vi "data processor main.vi"(11 "dataProcessor":T1) -> ()   [LabVIEW 2018]
uses:
  type defs/data processor data.ctl
  type defs/channelLimitControl.ctl
  type defs/limitActions.ctl
  supporting VIs/polymorphic VIs/de-queue for data processor.vi
  supporting VIs/polymorphic VIs/enqueue for file IO.vi
  supporting VIs/polymorphic VIs/release data processor queue.vi
types:
  T1 = typedef "data processor data.ctl" = cluster{"params":cluster{"controlFeedback":cluster{"butterflyValue":u16, "ballValue":u16, "massflow":u16, "pressureRatio":u16, "compSpeed":u16}, "DAQrate":enum16{"50 kHz", "25 kHz", "16.6 kHz", "12.5 kHz", "10 kHz", "8.33 kHz", "7.14 kHz", "6.25 kHz", "5.55 kHz", "5 kHz"}, "safetyChannels":cluster{"oilP":u16, "airP":u16, "water":u16, "channelLimit":T2[]}, "channelConfigPath":path}, "vars":cluster{"controlFeedback":cluster{"butterflyValue":u16, "ballValue":u16, "massflow":u16, "pressureRatio":u16, "compSpeed":u16}, "activeChannelNames":string[], "activeChannelUnits":string[], "offset trigger":bool, "offsets":dbl[], "activeChannelLimitIndex":u16[], "liveData":bool}}
  T2 = typedef "channelLimitControl.ctl" = cluster{"channelID":u16, "Enabled":bool, "warnValue":dbl, "limitValue":dbl, "Invert":bool, "limitAction":T3}
  T3 = typedef "limitActions.ctl" = enum16{"stop", "shutdown", "ignore"}
  T4 = typedef "Queues.ctl" = cluster{"messageHandler":refnum<queue>, "comms":refnum<queue>, "dataStream":refnum<queue>, "dataProcessor":refnum<queue>, "fileIO":refnum<queue>, "userInterface":refnum<queue>, "errors":refnum<queue>, "customCompressor":refnum<queue>}
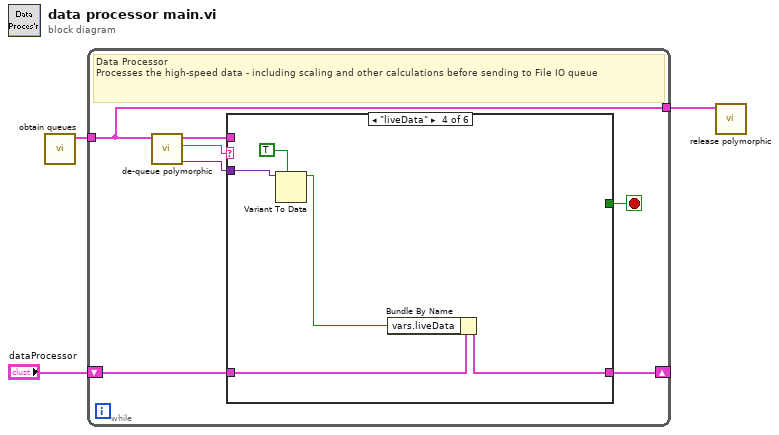
[diagram p0: block diagram]
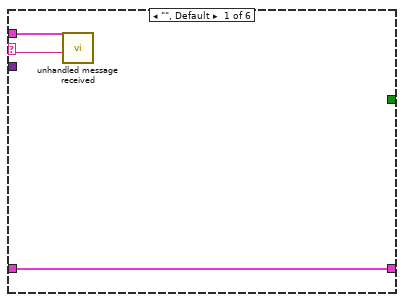
[diagram p2: hidden frame]
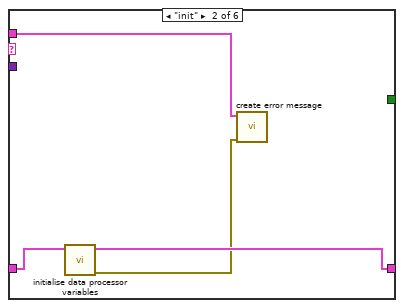
[diagram p3: hidden frame]
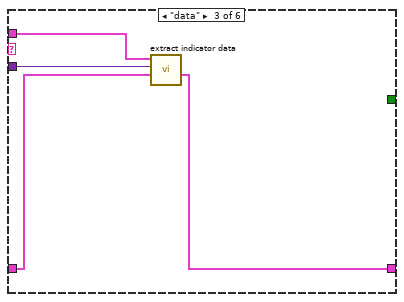
[diagram p4: hidden frame]
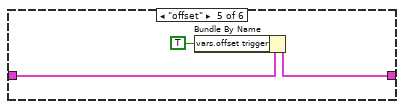
[diagram p5: hidden frame]
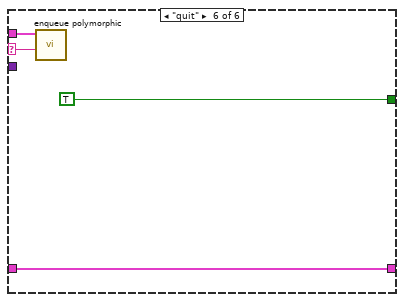
[diagram p6: hidden frame]
diagram:
  n1 = call "obtain queues.vi"() -> ("queues"=w2:T4)  [unwired: 11 in]
  n2 = while {
    tunnel: w2 -> [w6]
    tunnel: [w6] -> w1
    shift-right: [w5] -> _
    shift-left: "dataProcessor" -> [w4]
    stop <- w7 stop-if-true
    # "Data Processor\nProcesses the high-speed data - including scaling and other calculations before sending to File IO queue"
    n3 = call-poly "de-queue polymorphic.vi"("Queues"=w6) -> ("data"=w8:variant, "message"=w10:string, "Queues out"=w9:T4)  [unwired: 8 in]
    n4 = case shown="\"liveData\"" w10 {
      selector: w10 -> [w11 _ _ _ _ w32]
      tunnel: w9 -> [w12 w15 w19 _ _ w33]
      tunnel: w8 -> [_ _ w21 w25 _ _]
      tunnel: [_ _ _ _ _ TRUE] -> w7
      tunnel: [w13 w16 w18 w23 w28 w30] -> w5
      tunnel: w4 -> [w13 w17 w20 w26 w29 w30]
      frame "", Default {
        n5 = call "unhandled message received.vi"("unhandledMessage"=w11, "queues"=w12) -> ()  [unwired: 10 in]
      }
      frame "init" {
        n6 = call "initialise data processor variables.vi"("dataProcessor in"=w17) -> ("error out"=w14:errorcluster, "dataProcessor out"=w16:T1)  [unwired: 9 in]
        n7 = call "create error message.vi"("error in (no error)"=w14, "queues"=w15) -> ()  [unwired: 10 in]
      }
      frame "data" {
        n8 = call "extract indicator data.vi"("dataProcessor"=w20, "data in"=w21, "Queues in"=w19) -> ("dataProcessor out"=w18:T1)  [unwired: 7 in, 1 out]
      }
      frame "liveData" {
        n9 = Variant To Data(type=TRUE, Variant=w25) -> (data=w22:bool)  [unwired: 1 in, 1 out]
        n10 = Bundle By Name(cluster=w26, "vars.liveData"=w22) -> (w23:T1)
      }
      frame "offset" {
        n11 = Bundle By Name(cluster=w29, "vars.offset trigger"=TRUE) -> (w28:T1)
      }
      frame "quit" {
        n12 = call-poly "enqueue polymorphic.vi"("message"=w32, "Queues"=w33) -> ()  [unwired: 9 in, 1 out]
      }
    }
  }
  n13 = call-poly "release polymorphic.vi"("Queues"=w1) -> ()  [unwired: 11 in]
